vi "Do Write.vi"(8 "error in (no error)":errorcluster, 10 "Interface":refnum<class "Interface.lvclass">, 11 "Section in":refnum<class "Section.lvclass">) -> (0 "error out":errorcluster, 3 "Section out":refnum<class "Section.lvclass">, 4 "All Keys Found?":bool)   [LabVIEW 2012, in "Configuration.lvlib" / "Section.lvclass"]
doc: "Write keys/value pairs To Interface.\n\nThe baseclass implementation wirtes the item ClassPath to filebased configurations. Database othes other Interface are ignored. The need to care for themselfs.\n\nProtected dynamic dispatch VI to be overwritten by derived classes."
uses:
  Section.lvclass
  Interface/Interface.lvclass
  Config-File/Config-File.lvclass
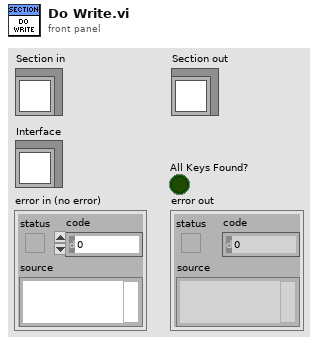
[diagram p1: front panel]
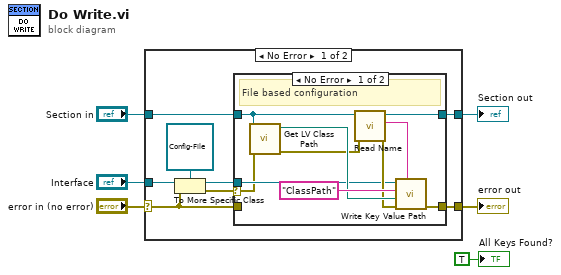
[diagram p0: block diagram]
diagram:
  n1 = case shown="No Error" "error in (no error)" {
    selector: "error in (no error)" -> [w7 w28]
    tunnel: [w12 w28] -> w5
    tunnel: [w14 w27] -> w3
    tunnel: "Section in" -> [w13 w27]
    tunnel: "Interface" -> [w11 _]
    frame No Error {
      n2 = To More Specific Class(target class=refnum<class "Config-File.lvclass"> refnum ("Configuration.lvlib:Config-File.lvclass"), reference=w11, error in=w7) -> (specific class reference=w10:refnum<class "Config-File.lvclass">, error out=w8:errorcluster)
      n3 = case shown="No Error" w8 {
        selector: w8 -> [w15 _]
        tunnel: [w24 w26] -> w14
        tunnel: w13 -> [w23 w26]
        tunnel: [w17 w25] -> w12
        tunnel: w10 -> [w16 _]
        tunnel: w7 -> [_ w25]
        frame No Error {
          # "File based configuration"
          n4 = call <vilib>:"Get LV Class Path.vi"("error in (no error)"=w15, "object"=w23) -> ("error out"=w19:errorcluster, "class path"=w20:path)  [unwired: 8 in]
          n5 = call "Read Name.vi"("error in (no error)"=w19, "Section in"=w23) -> ("error out"=w18:errorcluster, "Name"=w22:string, "Section out"=w24:refnum<class "Section.lvclass">)  [unwired: 7 in]
          n6 = call-dynamic "Write Key Value Path.vi"("Section Name"=w22, "error in (no error)"=w18, "Value"=w20, "Key Name"="ClassPath", "Interface in"=w16) -> ("error out"=w17:errorcluster)  [unwired: 4 in, 2 out]
        }
        frame Error {
          # "DB-based or somethiong else"
        }
      }
    }
    frame Error {
    }
  }
  "error out" <- w5
  "Section out" <- w3
  "All Keys Found?" <- TRUE ("All Keys Found?")
